vi "Init Error Log Filepath.vi"(8 "Error In":errorcluster, 10 "Error_Log_Setting":T1, 11 "Error Log Filepath Reference":refnum<vi>) -> (0 "Error Out":errorcluster)   [LabVIEW 2016, in "Error Manager.lvlib"]
doc: "Blank VI with error handling."
uses:
  Error Manager.lvlib
  Settings/Error_Log_Setting (enum).ctl
  Settings/Settings.lvclass
panel:
  # "Input\nInputs to the VI"
  # "Development\nControls or indicators that are useful for development or testing, but which are not outputs of the VI."
  # "Output\nOutputs of the VI"
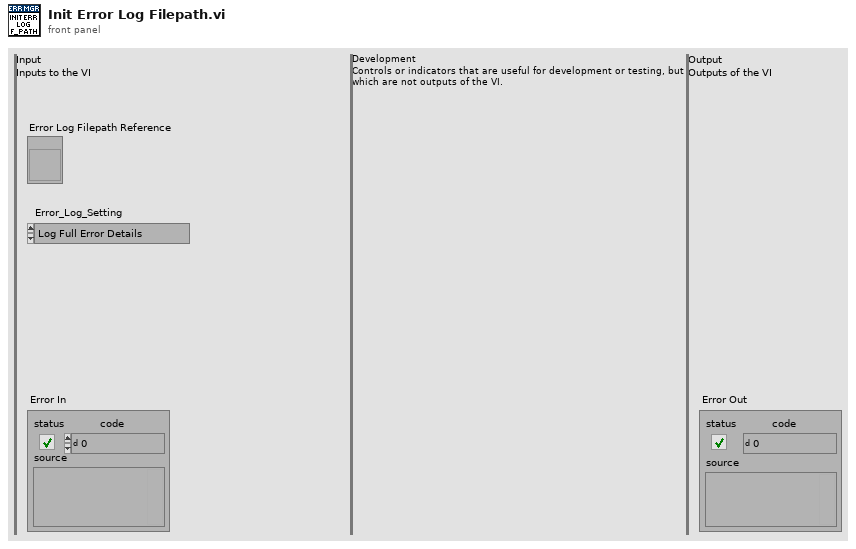
[diagram p1: front panel]
types:
  T1 = typedef "Error Manager.lvlib/Settings.lvclass/Error_Log_Setting (enum).ctl" = enum16{"Log Full Error Details", "Log Error Codes Only", "Do Not Log"}
  T2 = enum8{"Enabled", "Disabled", "Disabled and Grayed Out"}
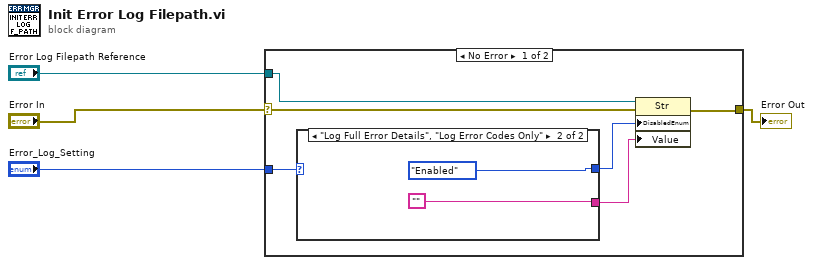
[diagram p0: block diagram]
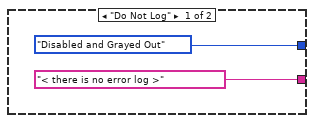
[diagram p2: hidden frame]
diagram:
  n1 = case shown="No Error" "Error In" {
    selector: "Error In" -> [w10 w15]
    tunnel: [w9 w15] -> w3
    tunnel: "Error Log Filepath Reference" -> [w8 _]
    tunnel: "Error_Log_Setting" -> [w7 _]
    frame No Error {
      n2 = case shown="\"Log Full Error Details\", \"Log Error Codes Only\"" w7 {
        tunnel: [T2."Disabled and Grayed Out" ("Disabled") T2."Enabled" ("Disabled")] -> w6
        tunnel: ["< there is no error log >" ("Boolean Text.Text") ""] -> w5
        frame "Do Not Log" {
        }
        frame "Log Full Error Details", "Log Error Codes Only" {
        }
      }
      n3 = property class="Str"(reference=w8, error in=w10, "DisabledEnum"=w6, "Value"=w5) -> (error out=w9:errorcluster)  [unwired: 1 out]
    }
    frame Error {
    }
  }
  "Error Out" <- w3
